vi "get_fav_colour.vi"() -> (4 "?":T2, 6 "Back out":T1, 8 "path":path)   [LabVIEW 2023]
doc: "Get the color from the user."
uses:
  custom_elements/fav_colorctl.ctl
  custom_elements/back_button.ctl
panel:
  in  "Back":T1
  in  "black":bool caption="BLACK"
  in  "blue":bool caption="BLUE"
  in  "green":bool caption="GREEN"
  in  "red":bool caption="RED"
  # "Select you favourite color"
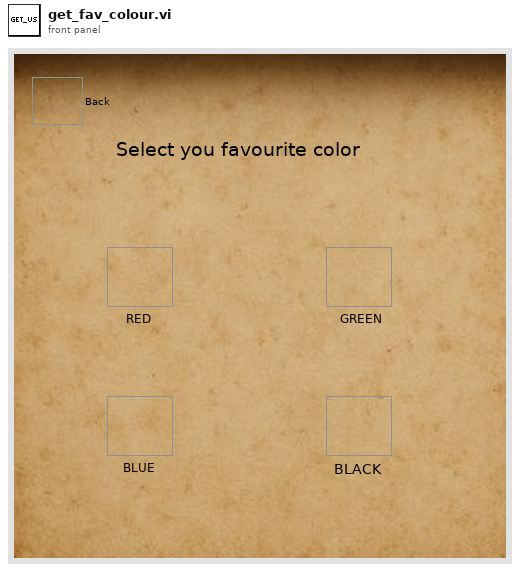
[diagram p1: front panel]
types:
  T1 = typedef "back_button.ctl" = bool
  T2 = typedef "fav_colorctl.ctl" = enum16{"black", "blue", "green", "red"}
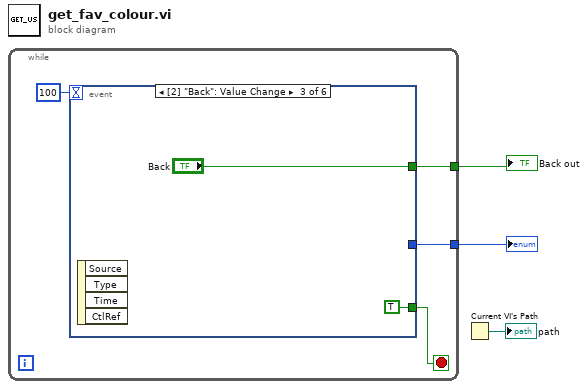
[diagram p0: block diagram]
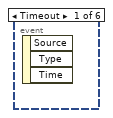
[diagram p2: hidden frame]
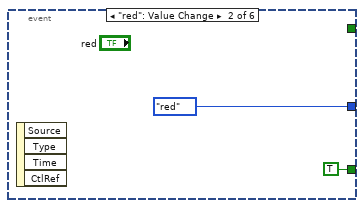
[diagram p3: hidden frame]
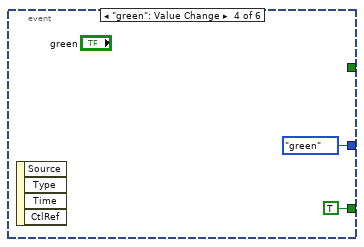
[diagram p4: hidden frame]
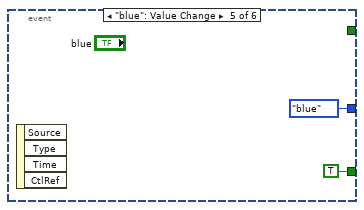
[diagram p5: hidden frame]
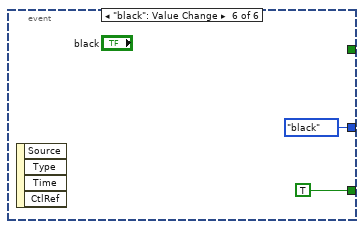
[diagram p6: hidden frame]
diagram:
  n1 = while {
    tunnel: [w6] -> w2
    tunnel: [w4] -> w1
    stop <- w5 stop-if-true
    n2 = event shown="[2] \"Back\": Value Change" {
      selector: _ -> [_ _ _ _ _ _]
      dyn-events: _ -> [_ _ _ _ _ _]
      timeout: 100 -> [_ _ _ _ _ _]
      tunnel: [_ fav_colorctl."red" _ fav_colorctl."green" fav_colorctl."blue" fav_colorctl."black"] -> w6
      tunnel: [_ TRUE TRUE TRUE TRUE TRUE] -> w5
      tunnel: [_ _ "Back" _ _ _] -> w4
      event Timeout {
        n3 = event-data() -> ()  [unwired: 1 in, 3 out]
      }
      event "red": Value Change {
        n4 = event-data() -> ()  [unwired: 1 in, 4 out]
      }
      event Value Change {
        n5 = event-data() -> ()  [unwired: 1 in, 4 out]
      }
      event "green": Value Change {
        n6 = event-data() -> ()  [unwired: 1 in, 4 out]
      }
      event "blue": Value Change {
        n7 = event-data() -> ()  [unwired: 1 in, 4 out]
      }
      event "black": Value Change {
        n8 = event-data() -> ()  [unwired: 1 in, 4 out]
      }
    }
  }
  "?" <- w2
  "Back out" <- w1
  n9 = Current VI's Path() -> (path=→"path":path)
